vi "XY Graph Update Plot.vi"(4 "Y Array":dbl[](array[numeric]), 6 "X Array":dbl[](array[numeric]), 8 "Error In":errorcluster, 9 "Plot":cluster{"X Array":dbl[], "Y Array":dbl[]}, 10 "Plot Idx":i32, 11 "XY Graph refnum":refnum<vi>) -> (0 "Error Out":errorcluster)   [LabVIEW 2019]
doc: "Update the Plot whose index is provided using either the Plot structure (first) or, if empty, the X and Y arrays.\nIf all are empty, then an empty plot is replacing the selected one."
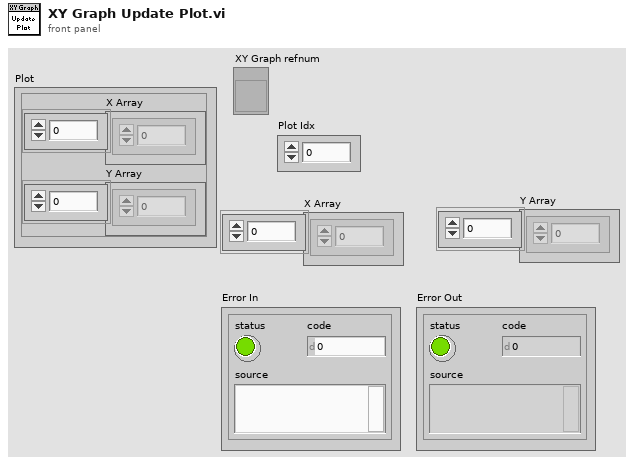
[diagram p1: front panel]
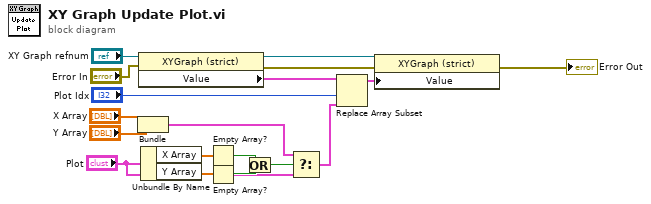
[diagram p0: block diagram]
diagram:
  n1 = Bundle("X Array"="X Array", "Y Array"="Y Array") -> (w3:cluster{"X Array":dbl[], "Y Array":dbl[]})  [unwired: 1 in]
  n2 = property class="XYGraph (strict)"(reference="XY Graph refnum", error in="Error In") -> (reference out=w14:refnum<vi>, error out=w13:errorcluster, "Value"=w17:cluster{"X Array":dbl[], "Y Array":dbl[]}[])
  n3 = Unbundle By Name("Plot") -> ("X Array"=w8:dbl[], "Y Array"=w7:dbl[])
  n4 = Empty Array?(array=w8) -> (empty?=w6:bool)
  n5 = Empty Array?(array=w7) -> (empty?=w5:bool)
  n6 = Or(x=w6, y=w5) -> (x .or. y?=w4:bool)
  n7 = Select(t=w3, s=w4, f="Plot") -> (s? t:f=w1:cluster{"X Array":dbl[], "Y Array":dbl[]})
  n8 = Replace Array Subset(array=w17, new element=w1, index="Plot Idx") -> (w12:cluster{"X Array":dbl[], "Y Array":dbl[]}[])
  n9 = property class="XYGraph (strict)"(reference=w14, error in=w13, "Value"=w12) -> (error out=→"Error Out":errorcluster)  [unwired: 1 out]
